vi "Motor_Actuation.vi"(8 "error in (no error)":errorcluster, 10 "LINX Resource in":T1, 11 "PID":ext) -> (0 "error out":errorcluster, 1 "Motor PWM":dbl=47.931426005026836, 2 "Saturated PD":dbl=47.931426005026836, 3 "LINX Resource":T1)   [LabVIEW 2021]
uses:
  <vilib>/MakerHub/LINX/Private/Type Defs/LINX Ref.ctl
  <vilib>/MakerHub/LINX/Private/Type Defs/Platform.ctl
  <vilib>/MakerHub/LINX/Private/Type Defs/Interface.ctl
  <vilib>/MakerHub/LINX/Private/Device/Type Defs/LINX Device Config.ctl
  <vilib>/MakerHub/LINX/Private/Device/Type Defs/TCP Config.ctl
  <vilib>/MakerHub/LINX/Private/Device/Type Defs/Channels.ctl
  <vilib>/MakerHub/LINX/Public/Peripherals/Digital/Digital Write 1 Chan.vi
  <vilib>/MakerHub/LINX/Public/Peripherals/PWM/PWM Set Duty Cycle 1 Chan.vi
  <vilib>/MakerHub/LINX/Public/Peripherals/Digital/Digital Write N Chans.vi
  <vilib>/MakerHub/LINX/Private/Local IO/LinxDigitalWrite.vi
  <vilib>/MakerHub/LINX/Public/Utilities/Check Channel.vi
  <vilib>/MakerHub/LINX/Private/Utilties/Generate Error.vi
  <vilib>/MakerHub/LINX/Public/Peripherals/PWM/PWM Set Duty Cycle N Chans.vi
  <vilib>/MakerHub/LINX/LMH-LINX.lvlib
  <vilib>/MakerHub/LINX/Private/Device/Device.lvlib
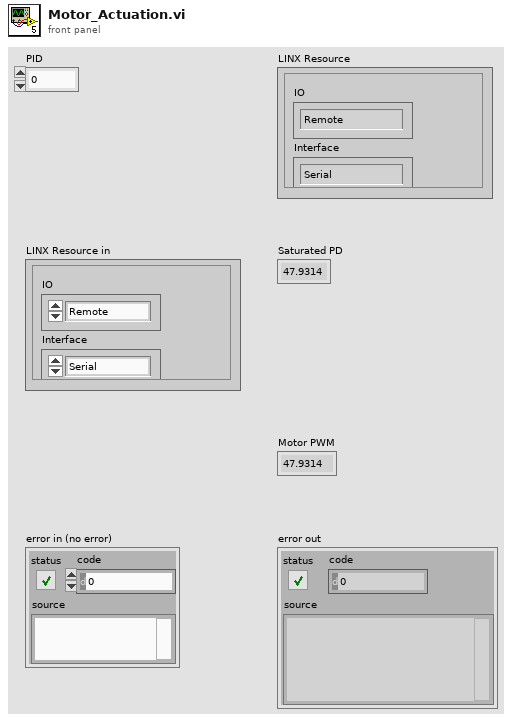
[diagram p1: front panel]
types:
  T1 = typedef "LMH-LINX.lvlib/LINX Ref.ctl" = cluster{"IO":T2, "Interface":T3, "LINX Device Config":T4}
  T2 = typedef "LMH-LINX.lvlib/Platform.ctl" = enum16{"Remote", "Local"}
  T3 = typedef "LMH-LINX.lvlib/Interface.ctl" = enum16{"Serial", "TCP"}
  T4 = typedef "LMH-LINX.lvlib/Device.lvlib/LINX Device Config.ctl" = cluster{"Interface":T3, "COM Port":refnum<visa-resource-name>, "TCP Configuration":T5, "Device Family":u8, "Device ID":u8, "Device Name":string, "TCP Ref":refnum<k5>, "Channels":T6}
  T5 = typedef "LMH-LINX.lvlib/Device.lvlib/TCP Config.ctl" = cluster{"IP Address":string, "Port":u16}
  T6 = typedef "LMH-LINX.lvlib/Channels.ctl" = cluster{"DI":u8[], "DO":u8[], "AI":u8[], "AO":u8[], "PWM":u8[], "QE":u8[], "UART":u8[], "I2C 2":u8[], "SPI":u8[], "CAN":u8[], "Servo":u8[], "AI Ref (V)":dbl, "AI Resolution (Bits)":u8, "AO Ref (V)":dbl, "AO Resolution (Bits)":u8}
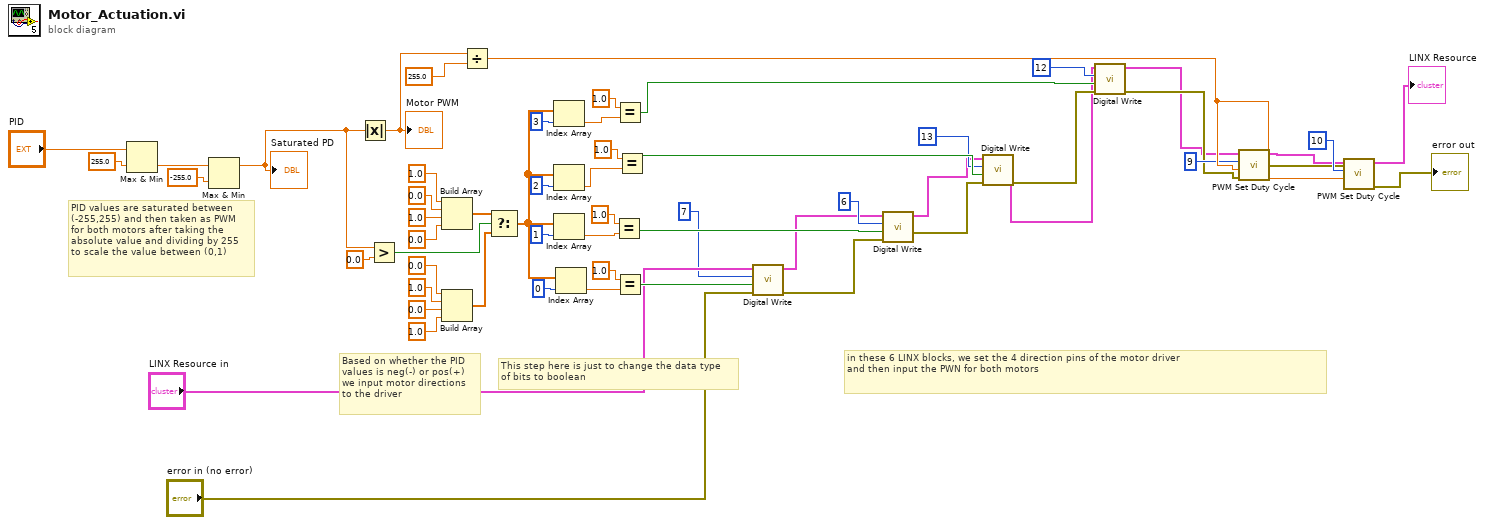
[diagram p0: block diagram]
diagram:
  # "in these 6 LINX blocks, we set the 4 direction pins of the motor driver\nand then input the PWN for both motors"
  # "This step here is just to change the data type \nof bits to boolean"
  # "Based on whether the PID\nvalues is neg(-) or pos(+)\nwe input motor directions\nto the driver"
  # "PID values are saturated between \n(-255,255) and then taken as PWM\nfor both motors after taking the\nabsolute value and dividing by 255\nto scale the value between (0,1)"
  n1 = Max & Min(x="PID", y=255.0) -> (min(x,y)=w22:ext)  [unwired: 1 out]
  n2 = Max & Min(x=w22, y=-255.0) -> (max(x,y)=w51:ext)  [unwired: 1 out]
  "Saturated PD" <- w51
  n3 = Absolute Value(x=w51) -> (abs(x)=w52:ext)
  "Motor PWM" <- w52
  n4 = Greater?(x=w51, y=0.0) -> (0:w25:bool)
  n5 = Build Array(1.0 ("element"), 0.0 ("element"), 1.0 ("element"), 0.0 ("element")) -> (w30:dbl[])
  n6 = Build Array(0.0 ("element"), 1.0 ("element"), 0.0 ("element"), 1.0 ("element")) -> (w35:dbl[])
  n7 = Divide(x=w52, y=255.0) -> (x/y=w55:ext)
  n8 = Select(t=w30, s=w25, f=w35) -> (s? t:f=w40:dbl[])
  n9 = Index Array(array=w40, index=3) -> (element=w48:dbl)
  n10 = Index Array(array=w40, index=2) -> (element=w47:dbl)
  n11 = Index Array(array=w40, index=1) -> (element=w46:dbl)
  n12 = Index Array(array=w40, index=0) -> (element=w41:dbl)
  n13 = Equal?(x=1.0, y=w46) -> (x = y?=w54:bool)
  n14 = Equal?(x=1.0, y=w48) -> (x = y?=w50:bool)
  n15 = Equal?(x=1.0, y=w41) -> (x = y?=w49:bool)
  n16 = Equal?(x=1.0, y=w47) -> (x = y?=w53:bool)
  n17 = call-poly <vilib>:"Digital Write.vi"("Error In"="error in (no error)", "Output Value"=w49, "DO Channel"=u8 7, "LINX Resource"="LINX Resource in") -> ("Error Out"=w7:errorcluster, "LINX Resource"=w1:T1)  [unwired: 6 in]
  n18 = call-poly <vilib>:"Digital Write.vi"("Error In"=w7, "Output Value"=w54, "DO Channel"=u8 6, "LINX Resource"=w1) -> ("Error Out"=w8:errorcluster, "LINX Resource"=w2:T1)  [unwired: 6 in]
  n19 = call-poly <vilib>:"Digital Write.vi"("Error In"=w8, "Output Value"=w53, "DO Channel"=u8 13, "LINX Resource"=w2) -> ("Error Out"=w9:errorcluster, "LINX Resource"=w3:T1)  [unwired: 6 in]
  n20 = call-poly <vilib>:"Digital Write.vi"("Error In"=w9, "Output Value"=w50, "DO Channel"=u8 12, "LINX Resource"=w3) -> ("Error Out"=w10:errorcluster, "LINX Resource"=w4:T1)  [unwired: 6 in]
  n21 = call-poly <vilib>:"PWM Set Duty Cycle.vi"("Error In"=w10, "Duty Cycle (0-1)"=w55, "PWM Channel"=u8 9, "LINX Resource"=w4) -> ("Error Out"=w11:errorcluster, "LINX Resource"=w5:T1)  [unwired: 6 in]
  n22 = call-poly <vilib>:"PWM Set Duty Cycle.vi"("Error In"=w11, "Duty Cycle (0-1)"=w55, "PWM Channel"=u8 10, "LINX Resource"=w5) -> ("Error Out"=→"error out":errorcluster, "LINX Resource"=→"LINX Resource":T1)  [unwired: 6 in]
